vi "AddWeightedImagesGreyscale.vi"(5 "B":dbl=0.5, 6 "C (Default: 0)":dbl, 7 "A":dbl=0.5, 8 "error in (no error)":errorcluster, 9 "Greyscale Destination":refnum<data-value>, 10 "Greyscale Image B":refnum<data-value>, 11 "Greyscale Image A":refnum<data-value>) -> (0 "error out":errorcluster, 3 "Greyscale Destination (Duplicate)":refnum<data-value>)   [LabVIEW 2020, in "g_ar_toolkit.image.lvlib"]
uses:
  g_ar_toolkit.image.lvlib
  <vilib>/Utility/error.llb/Error Cluster From Error Code.vi
  2e5e2c88-b721-4a80-abe1-d690325a547c.vi
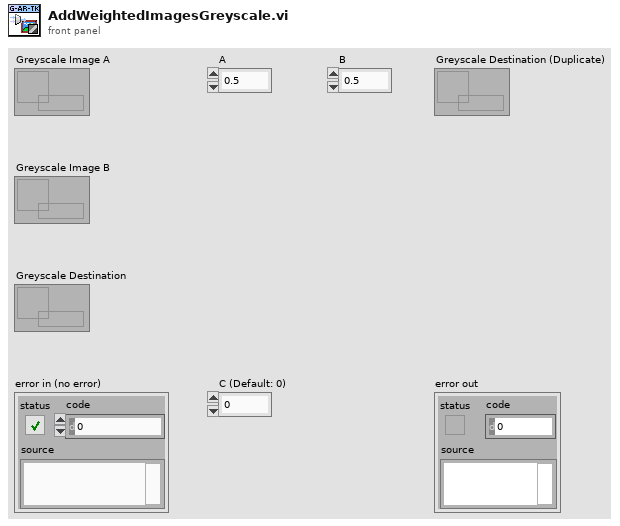
[diagram p1: front panel]
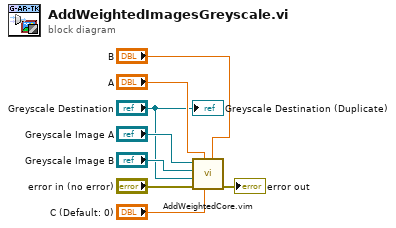
[diagram p0: block diagram]
diagram:
  n1 = call "AddWeightedCore.vim"(5:"B"="B", "C"="C (Default: 0)", 7:"A"="A", "error in (no error)"="error in (no error)", "Dst"="Greyscale Destination", 10:"B"="Greyscale Image B", 11:"A"="Greyscale Image A") -> ("error out"=→"error out":errorcluster)  [unwired: 4 in]
  "Greyscale Destination (Duplicate)" <- "Greyscale Destination"
